vi "Close.vi"(8 "error in (no error)":errorcluster, 11 "InfoService in":refnum<class "NodeStatus.lvclass">) -> (0 "error out":errorcluster)   [LabVIEW 2020, in "Vecto.lvlib" / "NodeStatus.lvclass"]
uses:
  NodeStatus.lvclass
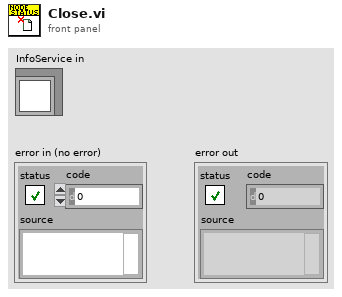
[diagram p1: front panel]
types:
  T1 = typedef "Vecto.lvlib/NodeStatus.lvclass/Incoming Events.ctl" = cluster{"Info Request":refnum<user-event>, "Update Task":refnum<user-event>, "Update Info":refnum<user-event>, "Close":refnum<user-event>}
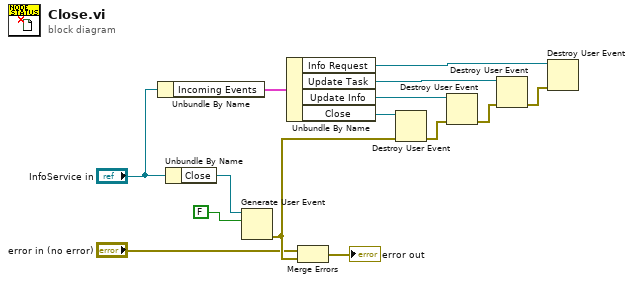
[diagram p0: block diagram]
diagram:
  n1 = Unbundle By Name("InfoService in") -> ("Incoming Events"=w11:T1)
  n2 = Unbundle By Name("InfoService in") -> ("Close"=w14:refnum<user-event>)
  n3 = Generate User Event(user event=w14, event data cluster=FALSE ("event data")) -> (error out=w9:errorcluster)  [unwired: 2 in, 1 out]
  n4 = Unbundle By Name(w11) -> ("Info Request"=w1:refnum<user-event>, "Update Task"=w3:refnum<user-event>, "Update Info"=w6:refnum<user-event>, "Close"=w10:refnum<user-event>)
  n5 = Merge Errors("error in (no error)", w9) -> (→"error out":errorcluster)
  n6 = Destroy User Event(user event=w10, error in=w9) -> (error out=w5:errorcluster)
  n7 = Destroy User Event(user event=w6, error in=w5) -> (error out=w2:errorcluster)
  n8 = Destroy User Event(user event=w3, error in=w2) -> (error out=w4:errorcluster)
  n9 = Destroy User Event(user event=w1, error in=w4) -> ()  [unwired: 1 out]
